vi "LVCAM Destroy.vi"(10 "Error":errorcluster, 11 "LVCAM Destroy in":refnum<class "LVCAM Destroy.lvclass">) -> ()   [LabVIEW 2021, in "LVCAM.lvlib" / "LVCAM Destroy.lvclass"]
uses:
  LVCAM Destroy.lvclass
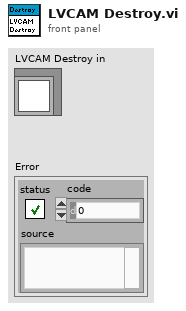
[diagram p1: front panel]
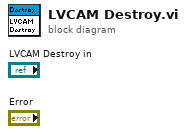
[diagram p0: block diagram]
diagram:
